vi "Launcher.vi"   [LabVIEW 2019]
uses:
  Calling Actor/Calling Actor.lvclass
  C:/Program Files (x86)/National Instruments/LabVIEW 2019/vi.lib/ActorFramework/Actor/Actor.lvclass
  <vilib>/ActorFramework/Actor/Actor.lvclass
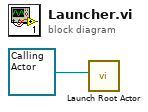
[diagram p0: block diagram]
diagram:
  n1 = call <vilib>:"Launch Root Actor.vi"("Actor"=refnum<class "Calling Actor.lvclass"> refnum ("Calling Actor.lvlib:Calling Actor.lvclass")) -> ()  [unwired: 9 in, 2 out]
